vi "Read TimeDomainFile.vi"(8 "error in":errorcluster, 11 "PAS in":refnum<class "PAS.lvclass">) -> (0 "error out":errorcluster, 2 "File Obs":refnum<class "File Observer.lvclass">, 3 "PAS out":refnum<class "PAS.lvclass">)   [LabVIEW 2015, in "PAS.lvclass"]
uses:
  PAS.lvclass
  File IO/Class/File Observer.lvclass
  PAS.lvclass/PAS.ctl
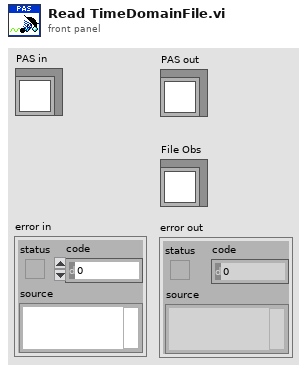
[diagram p1: front panel]
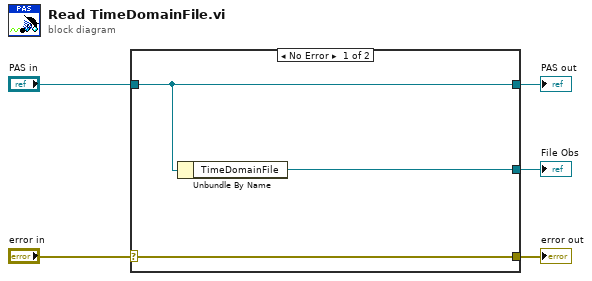
[diagram p0: block diagram]
diagram:
  n1 = case shown="No Error" "error in" {
    selector: "error in" -> [w8 w9]
    tunnel: [w8 w9] -> w4
    tunnel: [w7 w10] -> w2
    tunnel: "PAS in" -> [w7 w10]
    tunnel: [w6 _] -> w1
    frame No Error {
      n2 = Unbundle By Name(w7) -> ("TimeDomainFile"=w6:refnum<class "File Observer.lvclass">)
    }
    frame Error {
    }
  }
  "error out" <- w4
  "PAS out" <- w2
  "File Obs" <- w1
